vi "Scan and Shutter Control.vi"(9 "stop acquisition at\nFIFO overflow?":bool, 10 "fifo overflow in":bool, 11 "scan":bool) -> (1 "FIFO overflow":bool, 3 "scanning?":bool)   [LabVIEW 2010]
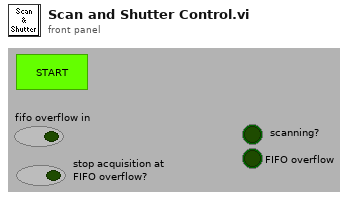
[diagram p1: front panel]
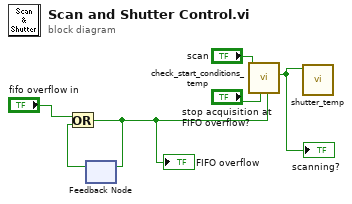
[diagram p0: block diagram]
diagram:
  n1 = feedback #1() -> (w2:bool)  [unwired: 1 in]
  n2 = Or(x="fifo overflow in", y=w2) -> (x .or. y?=w1:bool)
  "FIFO overflow" <- w1
  n3 = feedback-in #1(w1) -> ()
  n4 = call "check_start_conditions_temp.vi"("FIFO overflow?"=w1, "stop at FIFO overflow?"="stop acquisition at\nFIFO overflow?", "acquire"="scan") -> ("acquire?"=w4:bool)  [unwired: 8 in]
  "scanning?" <- w4
  n5 = call "shutter_temp.vi"("open?"=w4) -> ()  [unwired: 11 in]
